vi "createState.vi"(8 "error in (no error)":errorcluster, 10 "State:":T1, 11 "StateFactory in":refnum<class "StateFactory.lvclass">) -> (0 "error out":errorcluster, 2 "State.lvclass":refnum<class "State.lvclass">, 3 "StateFactory out":refnum<class "StateFactory.lvclass">)   [LabVIEW 2013, in "StateFactory.lvclass"]
uses:
  StateFactory.lvclass
  Typedefs/StateSelector.ctl
  State/State.lvclass
  States/EndingCycleState/EndingCycleState.lvclass
  States/FaultState/FaultState.lvclass
  States/InteractiveMotionState/InteractiveMotionState.lvclass
  States/MovingToNewForceState/MovingToNewForceState.lvclass
  States/OffState/OffState.lvclass
  States/PausingState/PausingState.lvclass
  States/StandbyState/StandbyState.lvclass
  States/StoppedState/StoppedState.lvclass
  Typedefs/M2AADTTypedefs.lvlib
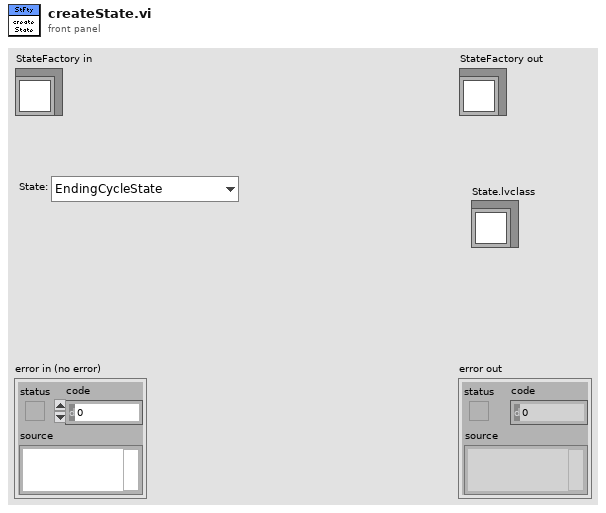
[diagram p1: front panel]
types:
  T1 = typedef "M2AADTTypedefs.lvlib/StateSelector.ctl" = enum16{"EndingCycleState", "FaultState", "InteractiveMotionState", "MovingToNewForceState", "OffState", "PausingState", "StandbyState", "StoppedState"}
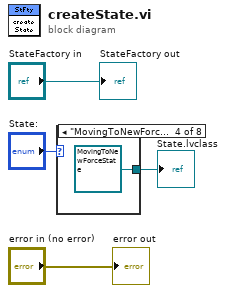
[diagram p0: block diagram]
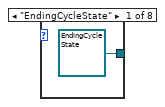
[diagram p2: hidden frame]
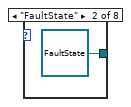
[diagram p3: hidden frame]
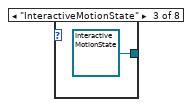
[diagram p4: hidden frame]
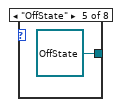
[diagram p5: hidden frame]
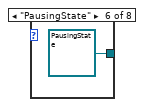
[diagram p6: hidden frame]
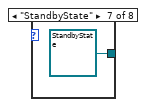
[diagram p7: hidden frame]
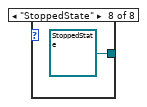
[diagram p8: hidden frame]
diagram:
  n1 = case shown="\"MovingToNewForceState\"" "State:" {
    tunnel: [refnum<class "EndingCycleState.lvclass"> refnum ("EndingCycleState.lvclass") refnum<class "FaultState.lvclass"> refnum ("FaultState.lvclass") refnum<class "InteractiveMotionState.lvclass"> refnum ("InteractiveMotionState.lvclass") refnum<class "MovingToNewForceState.lvclass"> refnum ("MovingToNewForceState.lvclass") refnum<class "OffState.lvclass"> refnum ("ShutdownState.lvclass") refnum<class "PausingState.lvclass"> refnum ("PausingState.lvclass") refnum<class "StandbyState.lvclass"> refnum ("StandbyState.lvclass") refnum<class "StoppedState.lvclass"> refnum ("StoppedState.lvclass")] -> w1
    frame "EndingCycleState" {
    }
    frame "FaultState" {
    }
    frame "InteractiveMotionState" {
    }
    frame "MovingToNewForceState" {
    }
    frame "OffState" {
    }
    frame "PausingState" {
    }
    frame "StandbyState" {
    }
    frame "StoppedState" {
    }
  }
  "State.lvclass" <- w1
  "error out" <- "error in (no error)"
  "StateFactory out" <- "StateFactory in"
